vi "Interpolate 2D Scattered (2D).vi"(6 "Yi":dbl[][](array[numeric]), 7 "method":i32(ring)=1 items=["nearest", "linear", "cubic", "biharmonic spline "], 8 "Xi":dbl[][](array[numeric]), 9 "Y":dbl[](array[numeric]), 10 "X":dbl[](array[numeric]), 11 "Z":dbl[](array[numeric])) -> (0 "error":i32, 3 "Zi":dbl[][](array[numeric]))   [LabVIEW 2017, in "NI_AAL_Interpolation.lvlib"]
doc: "Performs two-dimensional interpolation on scattered points."
uses:
  <vilib>/gmath/NI_AAL_Interpolation.lvlib
panel:
  # "Interpolate 2D Scattered (2D)"
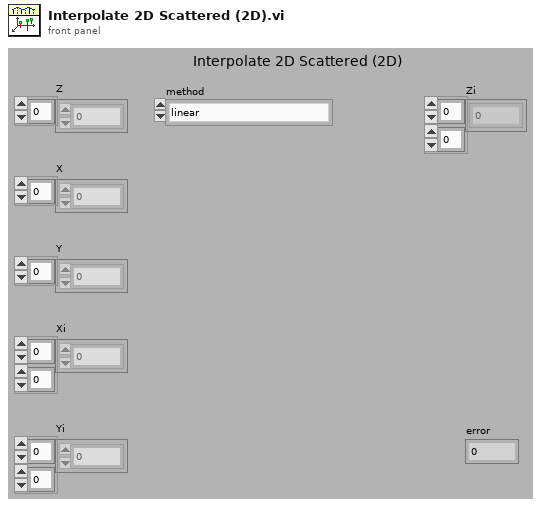
[diagram p1: front panel]
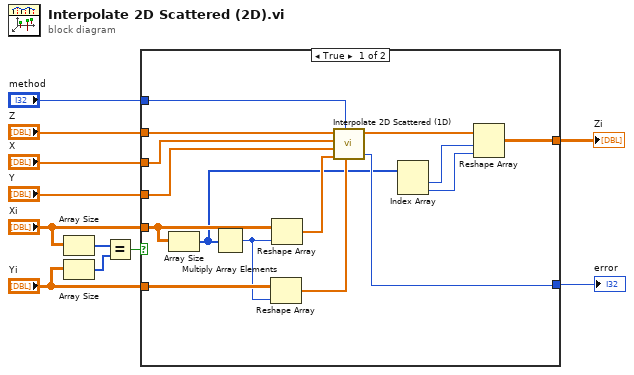
[diagram p0: block diagram]
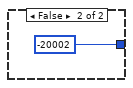
[diagram p2: hidden frame]
diagram:
  n1 = Array Size(array="Xi") -> (size(s)=w4:i32[])
  n2 = Array Size(array="Yi") -> (size(s)=w1:i32[])
  n3 = Equal?(x=w4, y=w1) -> (x = y?=w5:bool)
  n4 = case shown="True" w5 {
    tunnel: "Xi" -> [w14 _]
    tunnel: "Yi" -> [w26 _]
    tunnel: "Z" -> [w23 _]
    tunnel: "X" -> [w22 _]
    tunnel: "Y" -> [w21 _]
    tunnel: "method" -> [w20 _]
    tunnel: [w16 _] -> w7
    tunnel: [w15 -20002 ("error")] -> w6
    frame True {
      n5 = Array Size(array=w14) -> (size(s)=w12:i32[])
      n6 = Multiply Array Elements(1:w12) -> (0:w13:i32)
      n7 = Reshape Array(w26, w13) -> (w25:dbl[])
      n8 = Reshape Array(w14, w13) -> (w24:dbl[])
      n9 = call <vilib>:"Interpolate 2D Scattered (1D).vi"("Yi"=w25, "method"=w20, "Xi"=w24, "Y"=w21, "X"=w22, "Z"=w23) -> ("error"=w15:i32, "Zi"=w17:dbl[])  [unwired: 4 in]
      n10 = Index Array(array=w12) -> (element #1=w19:i32, element #2=w18:i32)  [unwired: 2 in]
      n11 = Reshape Array(w17, w19, w18) -> (w16:dbl[][])
    }
    frame False {
    }
  }
  "Zi" <- w7
  "error" <- w6
